vi "Litremeter top level.vi"() -> ()   [LabVIEW 2011]
panel:
  out "Sample DateTime":timestamp
  out "Time to fill (min)":dbl
  out "Fill rate":dbl(graph)
  out "Fill vol":dbl(graph)=1565.0
  in  "Tank capacity (L)":dbl=10000.0
  out "status":bool
  out "Tank fill (%)":dbl(slide) scale=0.0..100.0
  in  "Continuous measurement":bool
  out "status":bool
  out "Litres":dbl
  out "Pulses":u32
  in  "Single-shot measurement":bool
  in  "Default Litres / pulse cal. factor":dbl=1.0
  in  "Litres / pulse":dbl=1.0
  in  "Specify Litres / pulse cal. factor":bool
  in  "offset (L)":dbl
  in  "Specify fill offset":bool
  in  "Refresh rate (Hz)":dbl=10.0
  in  "stop":bool
  out "status":bool
  in  "Counter":tag="Dev2/ctr0"
  in  "Device":tag="Dev2"
  in  "Enable counter":bool
  # "Paul Nathan, 01/03/2012"
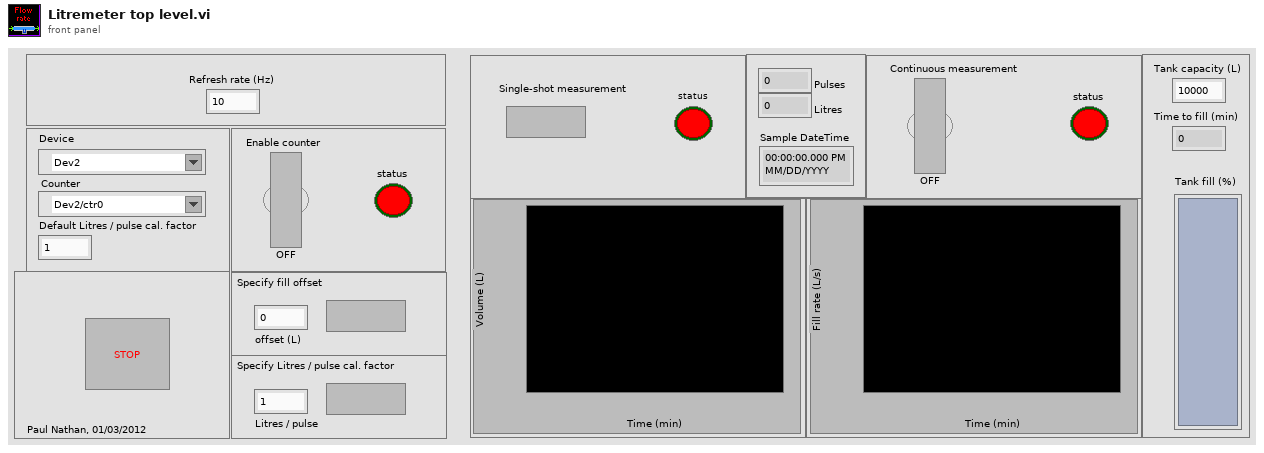
[diagram p1: front panel]
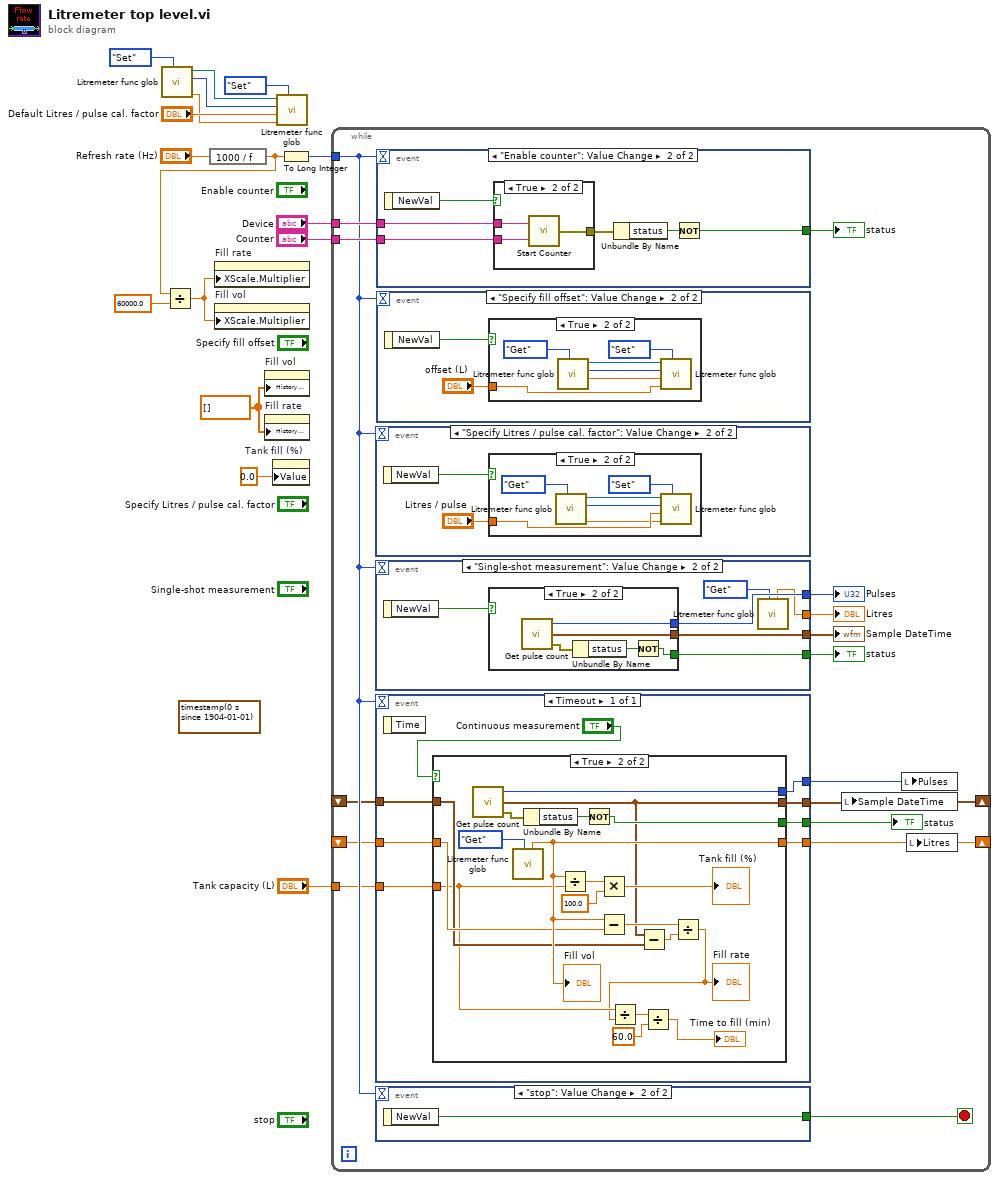
[diagram p0: block diagram]
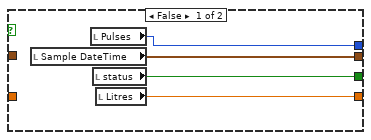
[diagram p2: hidden frame]
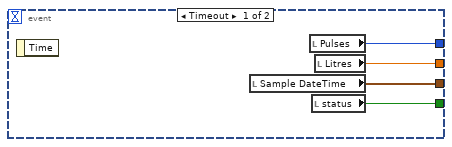
[diagram p3: hidden frame]
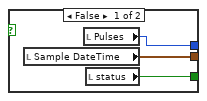
[diagram p4: hidden frame]
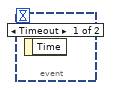
[diagram p5: hidden frame]
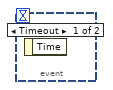
[diagram p7: hidden frame]
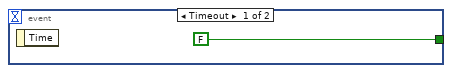
[diagram p9: hidden frame]
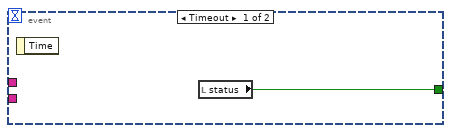
[diagram p10: hidden frame]
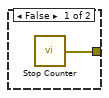
[diagram p11: hidden frame]
diagram:
  (unwired) timestamp(0 s since 1904-01-01)
  w5 = dbl[] [] ("History Data")
  n1 = call "Litremeter func glob.vi"("Action"=enum16{"Get", "Set"}."Set") -> ("Offset Litres out"=w10:dbl, "Pulse count out"=w9:u32, "Counter task out"=w8:refnum<k21>)  [unwired: 4 in, 2 out]
  n2 = expression code="1000 / f"("Refresh rate (Hz)") -> (w2:dbl)
  n3 = Divide(x=w2, y=60000.0) -> (x/y=w3:dbl)
  n4 = property on="Fill rate" class="WFChart (strict)"("XScale.Multiplier"=w3) -> ()  [unwired: 2 in, 2 out]
  n5 = property on="Fill vol" class="WFChart (strict)"("XScale.Multiplier"=w3) -> ()  [unwired: 2 in, 2 out]
  n6 = property on="Fill vol" class="WFChart (strict)"("History Data"=w5) -> ()  [unwired: 2 in, 2 out]
  n7 = property on="Fill rate" class="WFChart (strict)"("History Data"=w5) -> ()  [unwired: 2 in, 2 out]
  n8 = property on="Tank fill (%)" class="Slide (strict)"("Value"=0.0 ("Tank fill (%)")) -> ()  [unwired: 2 in, 2 out]
  n9 = call "Litremeter func glob.vi"("Action"=enum16{"Get", "Set"}."Set", "Offset Litres in"=w10, "Litres / pulse in"="Default Litres / pulse cal. factor", "Pulse count in"=w9, "Counter task in"=w8) -> ()  [unwired: 5 out]
  n10 = To Long Integer(number=w2) -> (32bit integer=w7:i32)
  n11 = while {
    tunnel: "Device" -> [w32]
    tunnel: "Counter" -> [w31]
    tunnel: w7 -> [w24]
    tunnel: "Tank capacity (L)" -> [w21]
    shift-right: [w20] -> _
    shift-left: _ -> [w19]
    shift-right: [w18] -> _
    shift-left: _ -> [w17]
    stop <- w30 stop-if-true
    n12 = event shown="[1] \"Specify Litres / pulse cal. factor\": Value Change" {
      selector: _ -> [_ _]
      dyn-events: _ -> [_ _]
      timeout: w24 -> [_ _]
      event Timeout {
        n13 = event-data() -> ()  [unwired: 1 in, 1 out]
      }
      event "Specify Litres / pulse cal. factor": Value Change {
        n14 = event-data() -> ("NewVal"=w83:bool)  [unwired: 1 in]
        n15 = case shown="True" w83 {
          tunnel: "Litres / pulse" -> [_ w87]
          frame False {
          }
          frame True {
            n16 = call "Litremeter func glob.vi"("Action"=enum16{"Get", "Set"}."Get") -> ("Offset Litres out"=w86:dbl, "Pulse count out"=w85:u32, "Counter task out"=w84:refnum<k21>)  [unwired: 4 in, 2 out]
            n17 = call "Litremeter func glob.vi"("Action"=enum16{"Get", "Set"}."Set", "Offset Litres in"=w86, "Litres / pulse in"=w87, "Pulse count in"=w85, "Counter task in"=w84) -> ()  [unwired: 5 out]
          }
        }
      }
    }
    n18 = event shown="[1] \"Single-shot measurement\": Value Change" {
      selector: _ -> [_ _]
      dyn-events: _ -> [_ _]
      timeout: w24 -> [_ _]
      tunnel: [w64 w69] -> w28
      tunnel: [w67 w72] -> w27
      tunnel: [w65 w71] -> w26
      tunnel: [w66 w68] -> w25
      event Timeout {
        n19 = event-data() -> ()  [unwired: 1 in, 1 out]
        n20 = local read "Sample DateTime"() -> (w65:timestamp)
        n21 = local read "Pulses"() -> (w67:u32)
        n22 = local read "status"() -> (w64:bool)
        n23 = local read "Litres"() -> (w66:dbl)
      }
      event "Single-shot measurement": Value Change {
        n24 = event-data() -> ("NewVal"=w73:bool)  [unwired: 1 in]
        n25 = case shown="True" w73 {
          tunnel: [w76 w81] -> w72
          tunnel: [w75 w80] -> w71
          tunnel: [w74 w77] -> w69
          frame False {
            n26 = local read "Sample DateTime"() -> (w75:timestamp)
            n27 = local read "Pulses"() -> (w76:u32)
            n28 = local read "status"() -> (w74:bool)
          }
          frame True {
            n29 = call "Get pulse count.vi"() -> ("Error"=w78:errorcluster, "Sample DateTime"=w80:timestamp, "Pulse count"=w81:u32)
            n30 = Unbundle By Name(w78) -> ("status"=w79:bool)
            n31 = Not(x=w79) -> (.not. x?=w77:bool)
          }
        }
        n32 = call "Litremeter func glob.vi"("Action"=enum16{"Get", "Set"}."Get") -> ("Total Litres (calc)"=w68:dbl)  [unwired: 4 in, 4 out]
      }
    }
    "Pulses" <- w27
    "Litres" <- w25
    "status" <- w28
    "Sample DateTime" <- w26
    n33 = event shown="[0] Timeout" {
      selector: _ -> [_]
      dyn-events: _ -> [_]
      timeout: w24 -> [_]
      tunnel: [w39] -> w23
      tunnel: [w38] -> w18
      tunnel: [w37] -> w22
      tunnel: [w36] -> w20
      tunnel: w21 -> [w35]
      tunnel: w19 -> [w34]
      tunnel: w17 -> [w33]
      event Timeout {
        n34 = event-data() -> ()  [unwired: 1 in, 1 out]
        n35 = case shown="True" "Continuous measurement" {
          tunnel: [w44 w63] -> w37
          tunnel: [w43 w50] -> w38
          tunnel: [w41 w60] -> w39
          tunnel: [w42 w55] -> w36
          tunnel: w35 -> [_ w49]
          tunnel: w34 -> [_ w54]
          tunnel: w33 -> [_ w52]
          frame False {
            n36 = local read "Sample DateTime"() -> (w43:timestamp)
            n37 = local read "Pulses"() -> (w44:u32)
            n38 = local read "status"() -> (w41:bool)
            n39 = local read "Litres"() -> (w42:dbl)
          }
          frame True {
            n40 = call "Get pulse count.vi"() -> ("Error"=w61:errorcluster, "Sample DateTime"=w50:timestamp, "Pulse count"=w63:u32)
            n41 = call "Litremeter func glob.vi"("Action"=enum16{"Get", "Set"}."Get") -> ("Total Litres (calc)"=w55:dbl)  [unwired: 4 in, 4 out]
            "Fill vol" <- w55
            n42 = Unbundle By Name(w61) -> ("status"=w62:bool)
            n43 = Divide(x=w55, y=w49) -> (x/y=w57:dbl)
            n44 = Not(x=w62) -> (.not. x?=w60:bool)
            n45 = Multiply(x=w57, y=100.0 ("x")) -> (x*y=→"Tank fill (%)":dbl)
            n46 = Subtract(x=w55, y=w54) -> (x-y=w53:dbl)
            n47 = Subtract(x=w50, y=w52) -> (x-y=w51:dbl)
            n48 = Divide(x=w53, y=w51) -> (x/y=w48:dbl)
            "Fill rate" <- w48
            n49 = Divide(x=w49, y=w48) -> (x/y=w47:dbl)
            n50 = Divide(x=w47, y=60.0) -> (x/y=→"Time to fill (min)":dbl)
          }
        }
      }
    }
    "status" <- w23
    n51 = event shown="[1] \"stop\": Value Change" {
      selector: _ -> [_ _]
      dyn-events: _ -> [_ _]
      timeout: w24 -> [_ _]
      tunnel: [FALSE ("NewVal") w99] -> w30
      event Timeout {
        n52 = event-data() -> ()  [unwired: 1 in, 1 out]
      }
      event "stop": Value Change {
        n53 = event-data() -> ("NewVal"=w99:bool)  [unwired: 1 in]
      }
    }
    n54 = event shown="[1] \"Enable counter\": Value Change" {
      selector: _ -> [_ _]
      dyn-events: _ -> [_ _]
      timeout: w24 -> [_ _]
      tunnel: w32 -> [_ w106]
      tunnel: w31 -> [_ w105]
      tunnel: [w100 w101] -> w29
      event Timeout {
        n55 = event-data() -> ()  [unwired: 1 in, 1 out]
        n56 = local read "status"() -> (w100:bool)
      }
      event "Enable counter": Value Change {
        n57 = event-data() -> ("NewVal"=w104:bool)  [unwired: 1 in]
        n58 = case shown="True" w104 {
          tunnel: w106 -> [_ w110]
          tunnel: w105 -> [_ w109]
          tunnel: [w107 w108] -> w102
          frame False {
            n59 = call "Stop Counter.vi"() -> ("Error"=w107:errorcluster)
          }
          frame True {
            n60 = call "Start Counter.vi"("Counter"=w109, "Device"=w110) -> ("Error"=w108:errorcluster)
          }
        }
        n61 = Unbundle By Name(w102) -> ("status"=w103:bool)
        n62 = Not(x=w103) -> (.not. x?=w101:bool)
      }
    }
    "status" <- w29
    n63 = event shown="[1] \"Specify fill offset\": Value Change" {
      selector: _ -> [_ _]
      dyn-events: _ -> [_ _]
      timeout: w24 -> [_ _]
      event Timeout {
        n64 = event-data() -> ()  [unwired: 1 in, 1 out]
      }
      event "Specify fill offset": Value Change {
        n65 = event-data() -> ("NewVal"=w91:bool)  [unwired: 1 in]
        n66 = case shown="True" w91 {
          tunnel: "offset (L)" -> [_ w93]
          frame False {
          }
          frame True {
            n67 = call "Litremeter func glob.vi"("Action"=enum16{"Get", "Set"}."Get") -> ("Litres / pulse out"=w94:dbl, "Pulse count out"=w92:u32, "Counter task out"=w95:refnum<k21>)  [unwired: 4 in, 2 out]
            n68 = call "Litremeter func glob.vi"("Action"=enum16{"Get", "Set"}."Set", "Offset Litres in"=w93, "Litres / pulse in"=w94, "Pulse count in"=w92, "Counter task in"=w95) -> ()  [unwired: 5 out]
          }
        }
      }
    }
    n69 = local write "Sample DateTime"(w18) -> ()
    n70 = local write "Pulses"(w22) -> ()
    n71 = local write "Litres"(w20) -> ()
  }
